vi "Error.vi"(10 "error in (no error)":errorcluster, 11 "PQ Connection in":refnum<class "PQ Connection.lvclass">) -> (2 "error out":errorcluster, 3 "PQ Connection out":refnum<class "PQ Connection.lvclass">)   [LabVIEW 2015, in "PQ Connection.lvclass"]
uses:
  PQ Connection.lvclass
  PQ Connection.lvclass/PQ Connection.ctl
  libpq.dll
panel:
  out "PQdb_ptr":u32
  out "PQerrorMessage_ptr":u32
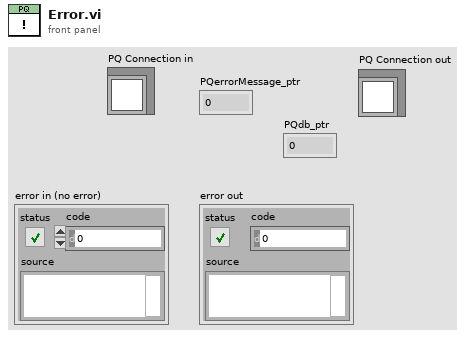
[diagram p1: front panel]
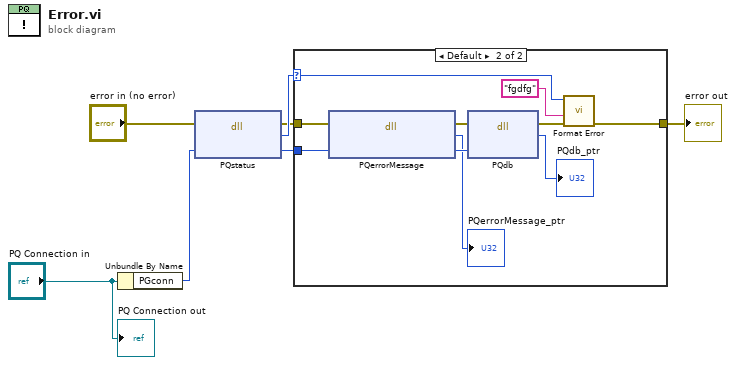
[diagram p0: block diagram]
diagram:
  n1 = Unbundle By Name("PQ Connection in") -> ("PGconn"=w6:u32)
  n2 = dll-call lib="C:/PQ/Connection/libpq.dll" fn="PQstatus"(error in="error in (no error)", "PGconn"=w6) -> (error out=w3:errorcluster, "PQstatus"=w5:u32, "PGconn"=w1:u32)  [unwired: 2 in, 1 out]
  n3 = case shown="Default" w5 {
    selector: w5 -> [_ w13]
    tunnel: w3 -> [w8 w18]
    tunnel: w1 -> [_ w17]
    tunnel: [w8 w9] -> w7
    frame 0 {
    }
    frame Default {
      n4 = dll-call lib="C:/PQ/Connection/libpq.dll" fn="PQerrorMessage"(error in=w18, "PGconn"=w17) -> (error out=w16:errorcluster, "PQerrorMessage_ptr"=→"PQerrorMessage_ptr":u32, "PGconn"=w15:u32)  [unwired: 2 in, 1 out]
      n5 = dll-call lib="C:/PQ/Connection/libpq.dll" fn="PQdb"(error in=w16, "PGconn"=w15) -> (error out=w10:errorcluster, "PQdb_ptr"=→"PQdb_ptr":u32)  [unwired: 3 in, 1 out]
      n6 = call "Format Error.vi"("error in (no error)"=w10, "Additional source description"="fgdfg", "error code"=w13) -> ("error out"=w9:errorcluster)  [unwired: 8 in]
    }
  }
  "error out" <- w7
  "PQ Connection out" <- "PQ Connection in"
